vi "Set Delay.vi"(6 "Delay (0) [s]":dbl format="%#_12g", 8 "error in (no error)":errorcluster, 9 "relative to (T0)":T1 items=["T0", "T1", "A", "B", "C", "D", "E", "F", "G", "H"], 10 "Channel (T0)":T1 items=["T0", "T1", "A", "B", "C", "D", "E", "F", "G", "H"], 11 "VISA resource name":refnum<visa-resource-name>) -> (0 "error out":errorcluster, 3 "VISA resource name out":refnum<visa-resource-name>, 4 "Device Errors":cluster{"code":i32, "Text":string}[](array[cluster]))   [LabVIEW 2014, in "Stanford Research DG645 - Driver.lvlib"]
doc: "Delay and Output Command: DLAY c,d,t\nInstrument Error Check\n\nSet the delay for Channel c to t (in seconds) relative to channel d."
uses:
  Stanford Research DG645 - Driver.lvlib
  Channel.ctl
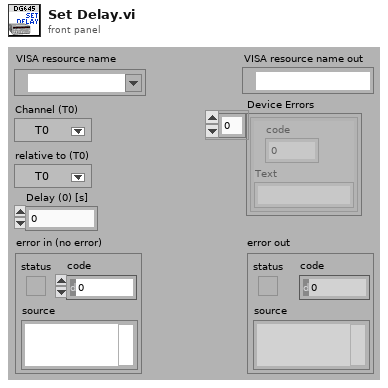
[diagram p1: front panel]
types:
  T1 = typedef "Stanford Research DG645 - Driver.lvlib/Channel.ctl" = i32
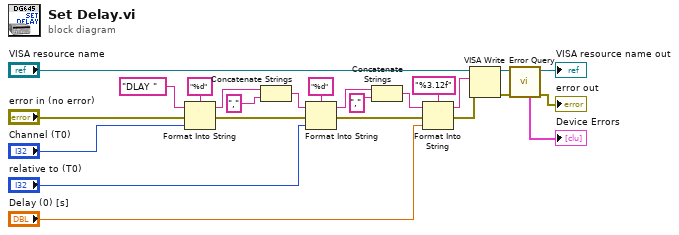
[diagram p0: block diagram]
diagram:
  n1 = Format Into String(format string="%d", initial string="DLAY " ("command"), error in="error in (no error)", "Channel (T0)") -> (resulting string=w21:string, error out=w22:errorcluster)
  n2 = Concatenate Strings(w21, "," ("command")) -> (w14:string)
  n3 = Format Into String(format string="%d", initial string=w14, error in=w22, "relative to (T0)") -> (resulting string=w16:string, error out=w17:errorcluster)
  n4 = Concatenate Strings(w16, "," ("command")) -> (w9:string)
  n5 = Format Into String(format string="%3.12f", initial string=w9, error in=w17, "Delay (0) [s]") -> (resulting string=w11:string, error out=w6:errorcluster)
  n6 = VISA Write(VISA resource name="VISA resource name", write buffer=w11, error in (no error)=w6) -> (VISA resource name out=w7:refnum<visa-resource-name>, error out=w3:errorcluster)  [unwired: 1 out]
  n7 = call "Error Query.vi"("error in (no error)"=w3, "VISA resource name"=w7) -> ("error out"=→"error out":errorcluster, "VISA resource name out"=→"VISA resource name out":refnum<visa-resource-name>, "Device Errors"=→"Device Errors":cluster{"code":i32, "Text":string}[])  [unwired: 7 in]
